vi "Write Build Name.vi"(8 "error in (no error)":errorcluster, 10 "Build Name":string, 11 "Build Job in":refnum<class "Build Job.lvclass">) -> (0 "error out":errorcluster, 3 "Build Job out":refnum<class "Build Job.lvclass">)   [LabVIEW 2014]
uses:
  Build Job.lvclass
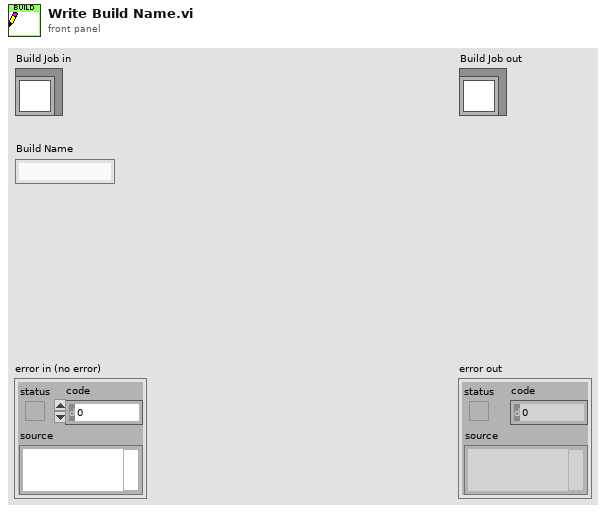
[diagram p1: front panel]
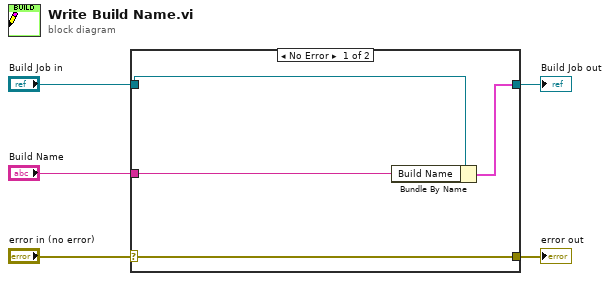
[diagram p0: block diagram]
diagram:
  n1 = case shown="No Error" "error in (no error)" {
    selector: "error in (no error)" -> [w9 w10]
    tunnel: [w9 w10] -> w4
    tunnel: [w7 w11] -> w2
    tunnel: "Build Job in" -> [w8 w11]
    tunnel: "Build Name" -> [w6 _]
    frame No Error {
      n2 = Bundle By Name(cluster=w8, "Build Name"=w6) -> (w7:cluster{})
    }
    frame Error {
    }
  }
  "error out" <- w4
  "Build Job out" <- w2
